vi "Initial Condition (DBL).vi"(2 "initialize":bool, 3 "initial condition":dbl format="%.2f", 5 "input point":dbl format="%.2f") -> (1 "output point":dbl format="%.2f")   [LabVIEW 2017, in "NI_AdvCtrl_nonlinear.lvlib"]
doc: "LabVIEW no longer supports this VI. You can obtain similar functionality by installing the LabVIEW Simulation Module.\n\nProduces a predefined initial condition immediately after the first call."
uses:
  <vilib>/addons/control/advanced/NI_AdvCtrl_nonlinear.lvlib
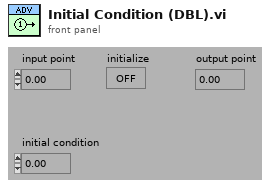
[diagram p1: front panel]
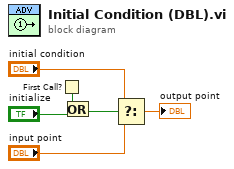
[diagram p0: block diagram]
diagram:
  n1 = First Call?() -> (First Call?: T/F=w3:bool)
  n2 = Or(x=w3, y="initialize") -> (x .or. y?=w1:bool)
  n3 = Select(t="initial condition", s=w1, f="input point") -> (s? t:f=→"output point":dbl)
